vi "Remove Empty Rows 2D.vi"(3 "Array In":string[][](array[string])) -> (1 "Array Out":string[][](array[string]))   [LabVIEW 2019]
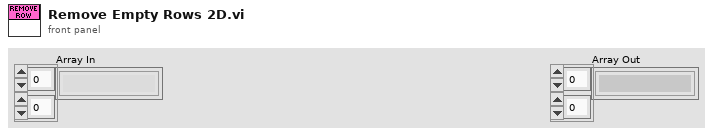
[diagram p1: front panel]
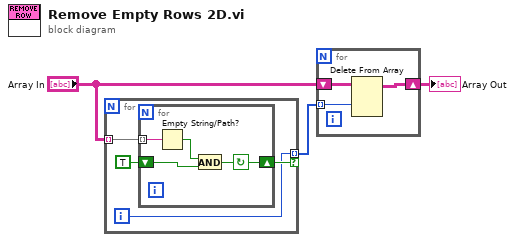
[diagram p0: block diagram]
diagram:
  n1 = for {
    tunnel: "Array In" -> [w7] mode=indexing
    tunnel: [w4] -> w2 mode=indexing if=w5
    i -> [w4]
    n2 = for {
      tunnel: w7 -> [w11] mode=indexing
      shift-right: [w8] -> w5
      shift-left: TRUE -> [w9]
      stop <- w8 continue-if-true
      n3 = Empty String/Path?(string/path=w11) -> (empty?=w10:bool)
      n4 = And(x=w10, y=w9) -> (x .and. y?=w8:bool)
    }
  }
  n5 = for {
    shift-right: [w13] -> w1
    shift-left: "Array In" -> [w14]
    tunnel: w2 -> [w12] mode=indexing
    n6 = Delete From Array(array=w14, index (row)=w12) -> (array with subset deleted=w13:string[][])  [unwired: 2 in, 1 out]
  }
  "Array Out" <- w1
